vi "Global QHnom.vi"() -> ()   [LabVIEW 2016]
panel:
  in  "q h nom":dbl[](array[numeric])
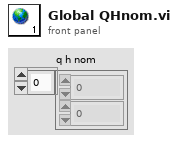
[diagram p1: front panel]
diagram:
